vi "Random Data.vi"() -> (0 "Data":dbl[](array[numeric]) format="%.2g")   [LabVIEW 2019]
panel:
  in  "Previous Data":dbl[](array[numeric]) format="%.2g"
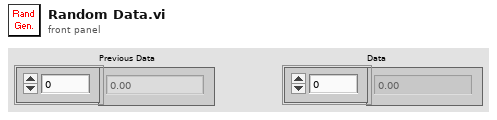
[diagram p1: front panel]
types:
  T1 = cluster{"TagId":string, "TagName":string, "TagType":string, "PhysicalChannel":tag, "Vmin":dbl, "Vmax":dbl, "Unit":string, "EUmin":dbl, "EUmax":dbl}[]
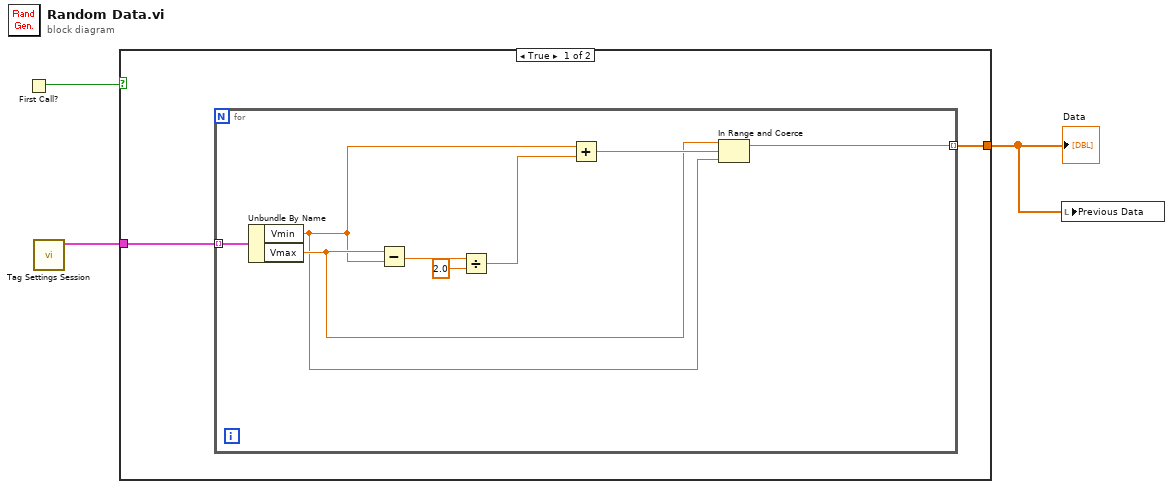
[diagram p0: block diagram]
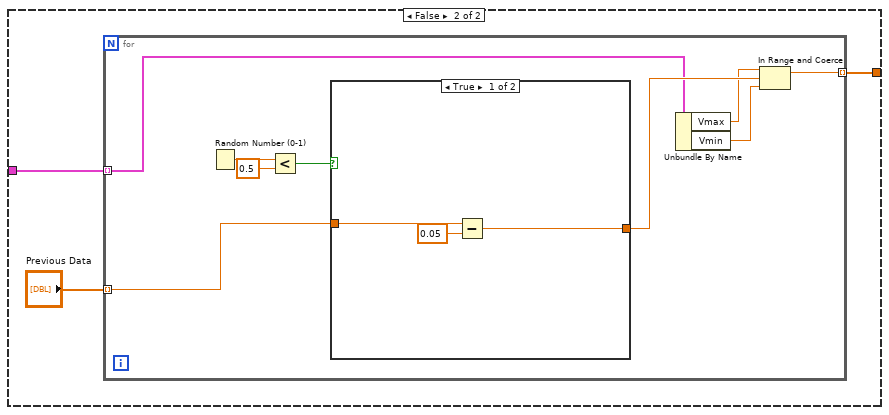
[diagram p2: hidden frame]
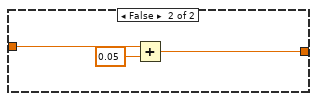
[diagram p3: hidden frame]
diagram:
  n1 = First Call?() -> (First Call?: T/F=w2:bool)
  n2 = call "Tag Settings Session.vi"() -> ("Tag Settings"=w1:T1)  [unwired: 10 in, 1 out]
  n3 = case shown="True" w2 {
    tunnel: w1 -> [w5 w16]
    tunnel: [w4 w15] -> w3
    frame True {
      n4 = for {
        tunnel: w5 -> [w12] mode=indexing
        tunnel: [w11] -> w4 mode=indexing
        n5 = Unbundle By Name(w12) -> ("Vmin"=w9:dbl, "Vmax"=w10:dbl)
        n6 = Subtract(x=w10, y=w9) -> (x-y=w8:dbl)
        n7 = Divide(x=w8, y=2.0) -> (x/y=w6:dbl)
        n8 = Add(x=w9, y=w6) -> (x+y=w13:dbl)
        n9 = In Range and Coerce(upper limit=w10, x=w13, lower limit=w9) -> (coerced(x)=w11:dbl)  [unwired: 1 out]
      }
    }
    frame False {
      n10 = for {
        tunnel: w16 -> [w19] mode=indexing
        tunnel: [w25] -> w15 mode=indexing
        tunnel: "Previous Data" -> [w22] mode=indexing
        n11 = Random Number (0-1)() -> (number: 0 to 1=w24:dbl)
        n12 = Less?(x=w24, y=0.5) -> (x < y?=w21:bool)
        n13 = case shown="True" w21 {
          tunnel: w22 -> [w28 w31]
          tunnel: [w26 w29] -> w20
          frame True {
            n14 = Subtract(x=w28, y=0.05) -> (x-y=w26:dbl)
          }
          frame False {
            n15 = Add(x=w31, y=0.05) -> (x+y=w29:dbl)
          }
        }
        n16 = Unbundle By Name(w19) -> ("Vmax"=w18:dbl, "Vmin"=w17:dbl)
        n17 = In Range and Coerce(upper limit=w18, x=w20, lower limit=w17) -> (coerced(x)=w25:dbl)  [unwired: 1 out]
      }
    }
  }
  "Data" <- w3
  n18 = local write "Previous Data"(w3) -> ()
